vi "Read PlatMods.vi"(8 "error in (no error)":errorcluster, 11 "ControlKeyDownMsg in":refnum<class "VIKeyDownMsg.lvclass">) -> (0 "error out":errorcluster, 2 "PlatMods":T1, 3 "ControlKeyDownMsg out":refnum<class "VIKeyDownMsg.lvclass">)   [LabVIEW 2020, in "ActorEvents.lvlib" / "VIKeyDownMsg.lvclass"]
uses:
  VIKeyDownMsg.lvclass
  VIKeyDownMsg.lvclass/VIKeyDownMsg.ctl
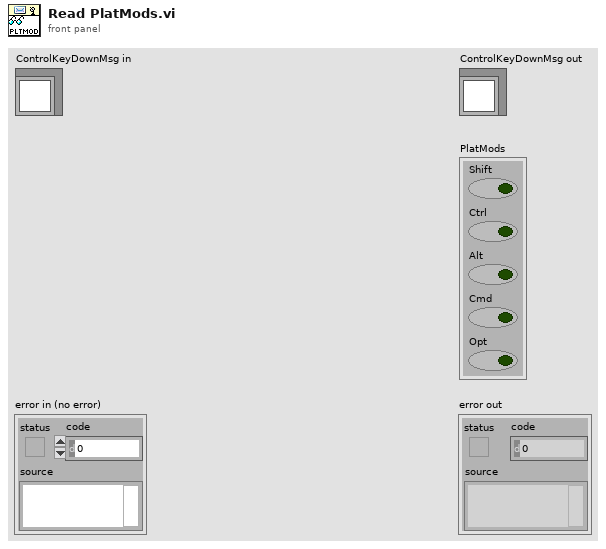
[diagram p1: front panel]
types:
  T1 = cluster{"Shift":bool, "Ctrl":bool, "Alt":bool, "Cmd":bool, "Opt":bool}
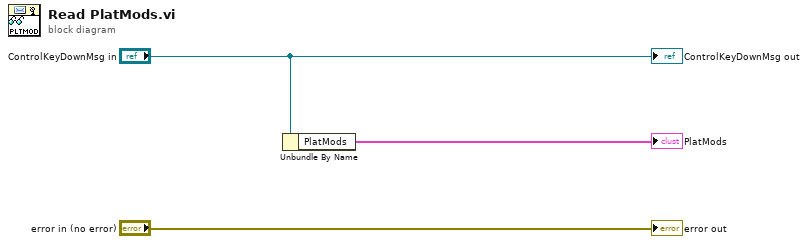
[diagram p0: block diagram]
diagram:
  n1 = Unbundle By Name("ControlKeyDownMsg in") -> ("PlatMods"=→"PlatMods":T1)
  "error out" <- "error in (no error)"
  "ControlKeyDownMsg out" <- "ControlKeyDownMsg in"
